vi "Write Data DVR.vi"(8 "error in (no error)":errorcluster, 10 "Data DVR":refnum<data-value>, 11 "cPAS Data DVR in":refnum<class "cPAS Data DVR.lvclass">) -> (0 "error out":errorcluster, 3 "cPAS Data DVR out":refnum<class "cPAS Data DVR.lvclass">)   [LabVIEW 2015, in "cPAS Data DVR.lvclass"]
uses:
  cPAS Data DVR.lvclass
  Reusable/Data/Data.lvclass
  cPAS Data DVR.lvclass/cPAS Data DVR.ctl
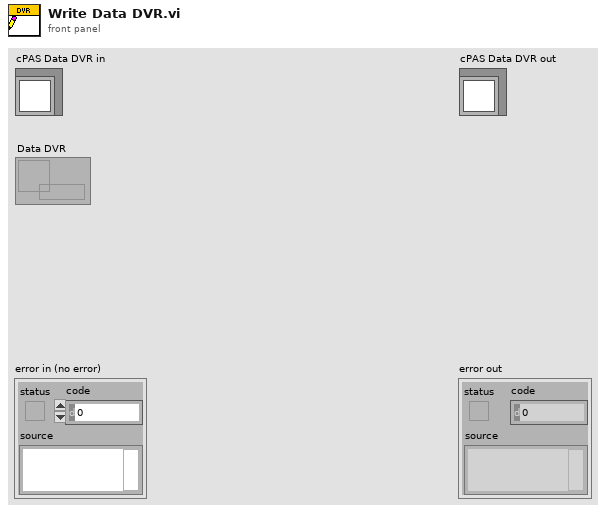
[diagram p1: front panel]
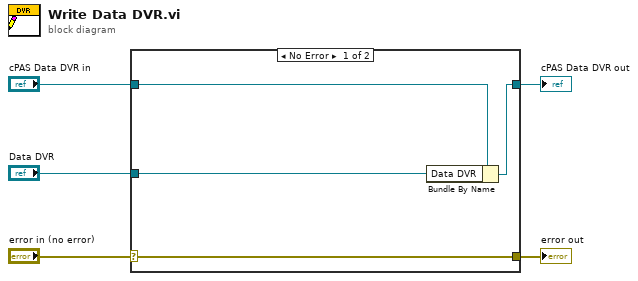
[diagram p0: block diagram]
diagram:
  n1 = case shown="No Error" "error in (no error)" {
    selector: "error in (no error)" -> [w9 w10]
    tunnel: [w9 w10] -> w4
    tunnel: [w7 w11] -> w2
    tunnel: "cPAS Data DVR in" -> [w8 w11]
    tunnel: "Data DVR" -> [w6 _]
    frame No Error {
      n2 = Bundle By Name(cluster=w8, "Data DVR"=w6) -> (w7:refnum<class "cPAS Data DVR.lvclass">)
    }
    frame Error {
    }
  }
  "error out" <- w4
  "cPAS Data DVR out" <- w2
